vi "Flanger.vi"(8 "error in (no error)":errorcluster, 10 "Audio Data In":dbl[][](array[numeric]), 11 "Effect in":refnum<class "Effect.lvclass">) -> (0 "error out":errorcluster, 2 "Audio Data Out":dbl[][](array[numeric]), 3 "Effect out":refnum<class "Effect.lvclass">)   [LabVIEW 2018, in "Effect.lvclass"]
uses:
  Effect.lvclass
  Effect.lvclass/Effect.ctl
  <vilib>/ptbypt/NI_PtbyPt.lvlib
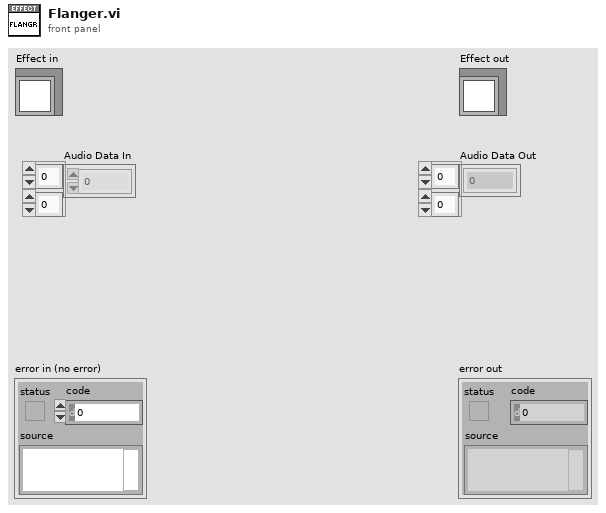
[diagram p1: front panel]
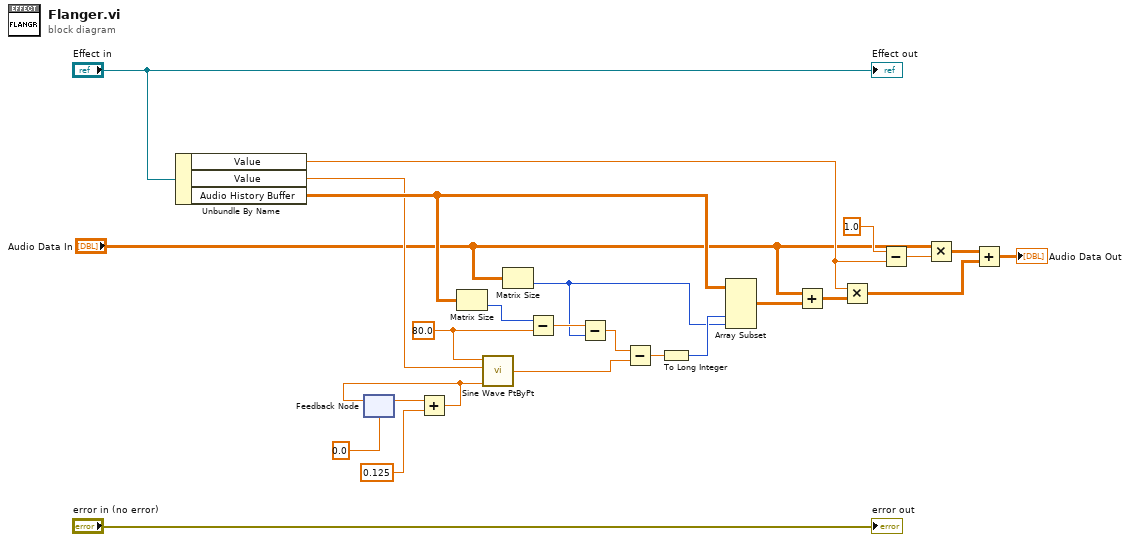
[diagram p0: block diagram]
diagram:
  w13 = 80.0 ("Delay")
  n1 = Unbundle By Name("Effect in") -> ("Value"=w3:dbl, "Value"=w4:dbl, "Audio History Buffer"=w5:dbl[][])
  n2 = feedback #1(0.0) -> (w16:dbl)
  n3 = Add(x=w16, y=0.125) -> (x+y=w18:dbl)
  n4 = feedback-in #1(w18) -> ()
  n5 = Matrix Size(0:w5) -> (2:w7:i32)  [unwired: 1 out]
  n6 = call <vilib>:"Sine Wave PtByPt.vi"("time"=w18, "frequency"=w4, "amplitude"=w13) -> ("sine wave"=w10:dbl)  [unwired: 1 in]
  n7 = Matrix Size(0:"Audio Data In") -> (2:w8:i32)  [unwired: 1 out]
  n8 = Subtract(x=w7, y=w13) -> (x-y=w14:dbl)
  n9 = Subtract(x=w14, y=w8) -> (x-y=w15:dbl)
  n10 = Subtract(x=w15, y=w10) -> (x-y=w11:dbl)
  n11 = To Long Integer(number=w11) -> (32bit integer=w12:i32)
  n12 = Array Subset(array=w5, index (col)=w12, length (col)=w8) -> (w24:dbl[][])  [unwired: 2 in]
  n13 = Add(x="Audio Data In", y=w24) -> (x+y=w19:dbl[][])
  n14 = Multiply(x=w3, y=w19) -> (x*y=w23:dbl[][])
  n15 = Subtract(x=1.0, y=w3) -> (x-y=w21:dbl)
  n16 = Multiply(x="Audio Data In", y=w21) -> (x*y=w22:dbl[][])
  n17 = Add(x=w22, y=w23) -> (x+y=→"Audio Data Out":dbl[][])
  "error out" <- "error in (no error)"
  "Effect out" <- "Effect in"
